vi "Solve1.vi"(8 "Error In":errorcluster, 11 "object in":refnum<class "2024_11.lvclass">) -> (0 "Error Out":errorcluster, 2 "Result":u64, 3 "object out":refnum<class "2024_11.lvclass">)   [LabVIEW 2023, in "2024_11.lvclass"]
uses:
  2024_11.lvclass
  2024_11.lvclass/2024_11.ctl
panel:
  out "x-y":u32
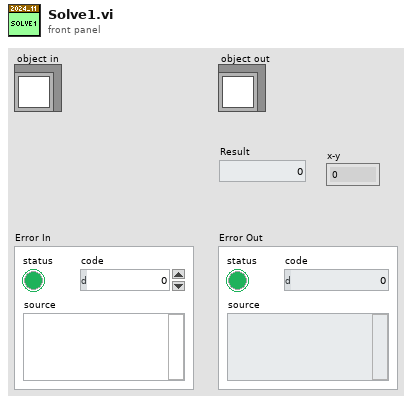
[diagram p1: front panel]
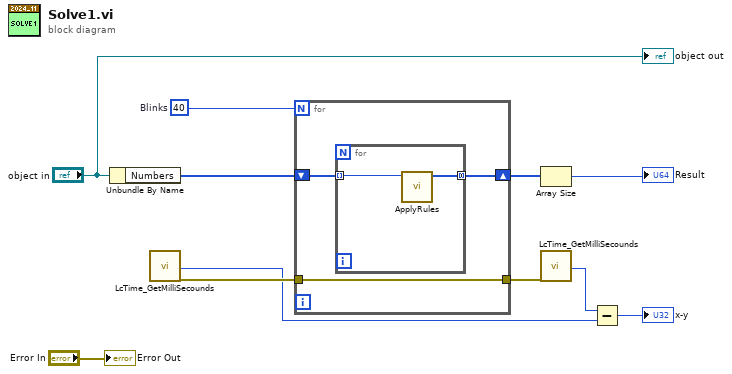
[diagram p0: block diagram]
diagram:
  w1 = 40  # Blinks
  n1 = Unbundle By Name("object in") -> ("Numbers"=w9:u64[])
  n2 = call <userlib>:"LcTime_GetMilliSecounds.vi"() -> ("msValue"=w3:u32, "error out"=w5:errorcluster)  [unwired: 18 in]
  n3 = for {
    N: w1 -> [_]
    shift-right: [w13] -> w8
    shift-left: w9 -> [w14]
    tunnel: [w12] -> w6
    tunnel: w5 -> [w12]
    n4 = for {
      tunnel: w14 -> [w15] mode=indexing
      tunnel: [w16] -> w13 mode=concatenating
      n5 = call "ApplyRules.vi"("Numeric"=w15) -> ("Array"=w16:u64[])  [unwired: 9 in, 1 out]
    }
  }
  n6 = Array Size(array=w8) -> (size(s)=→"Result":i32)
  n7 = call <userlib>:"LcTime_GetMilliSecounds.vi"("error in (no error)"=w6) -> ("msValue"=w4:u32)  [unwired: 17 in, 1 out]
  n8 = Subtract(x=w4, y=w3) -> (x-y=→"x-y":u32)
  "Error Out" <- "Error In"
  "object out" <- "object in"
